vi "Host - 2954 - 6592R Tx Streaming.vi"() -> ()   [LabVIEW 2018, in "Stream-2954-6592R.lvlib"]
uses:
  Stream-2954-6592R.lvlib
  <vilib>/userDefined/Silver/nirio_resource_slv.ctl
  TypeDefs/USRP Configuration.ctl
  TypeDefs/Playback Options.ctl
  TypeDefs/TDMS read.ctl
  TDMS Raw to Channels/Previewed Channel - Enum.ctl
  TypeDefs/Tx Config.ctl
  2954/SubVIs/Start Trigger.ctl
  <instrlib>/niUsrpRio/Config/v1/Host/Public/niUsrpRio Session.ctl
  <instrlib>/_niInstr/Register Bus/v0/Host/Public/Register Bus Session.ctl
  <instrlib>/_niInstr/Register Bus/v0/Host/Private/Session Data.ctl
  <instrlib>/niUsrpRio/Config/v1/Host/Private/DB Queue Reference.ctl
  <instrlib>/niUsrpRio/Config/v1/Host/Private/Daughterboard Data.ctl
  <instrlib>/niUsrpRio/Config/v1/Host/Private/ATR state data.ctl
  <instrlib>/niUsrpRio/Config/v1/Host/Private/Antenna Configuration.ctl
  <instrlib>/niUsrpRio/Config/v1/Host/Private/CPLD Power Mode.ctl
  <instrlib>/niUsrpRio/Config/v1/Host/Public/EEPROM Header.ctl
  <instrlib>/niUsrpRio/Config/v1/Host/Public/EEPROM Device Data Header.ctl
  <instrlib>/niUsrpRio/Config/v1/Host/Public/EEPROM Characterization Header.ctl
  <instrlib>/niUsrpRio/Config/v1/Host/Public/Characterization Data.ctl
  <instrlib>/niUsrpRio/Config/v1/Host/Public/IQ Imbalance.ctl
  TypeDefs/Rx Config.ctl
  TypeDefs/States.ctl
  <vilib>/FPGAPlugInAG/Dynamic/niLvFpga_Close_Dynamic.vi
  <vilib>/rvi/interface/nirviCloseFPGA/nirviCloseFPGA.xnode
  <instrlib>/niUsrpRio/Config/v1/Host/niUsrpRio Config v1 Host.lvlib
  <instrlib>/_niInstr/Register Bus/v0/Host/niInstr Register Bus v0 Host.lvlib
panel:
  out "Generating":bool
  in  "Tab Control":enum32{"Settings", "Debug"}(tab)
  in  "Playback Options":T1={"Infinite Generation"=FALSE, "max asynch. reads"=8, "Samples per Write"=14000000, "chunks"=8, "disable buffering?"=TRUE} {"chunks" format="%.0p"; "Samples per Write" format="%.3p"}
  in  "TDMS file paths":path[](array[path])=[path "R:/USRP_recording_ch1.tdms", path "R:/USRP_recording_ch0.tdms"]
  out "Actual FIFO Depths":u32[][](array[numeric])=[[112000000, 112000000]] format="%.3p"
  out "Underflow":bool
  out "tx.number of fifo underflows":u32[](array[numeric])
  in  "tx config":T2={"rf enable 0"=TRUE, "rf config 0"={"antenna"="TX1", "frequency"=2000000000.0, "lo frequency"=-1.0, "level"=0.0}, "rf enable 1"=TRUE, "rf config 1"={"antenna"="TX1", "frequency"=2000000000.0, "lo frequency"=-1.0, "level"=0.0}, "transfer mode"=enum."Continuous", "sample rate"=200000000.0, "start trigger"=enum."Software"} {"sample rate" format="%#.3pS/s"; "rf config 0"."level" format="%#_gdBm"; "rf config 0"."lo frequency" format="%#.3pHz"; "rf config 0"."frequency" format="%#.3pHz"; "rf config 1"."level" format="%#_gdBm"; "rf config 1"."lo frequency" format="%#.3pHz"; "rf config 1"."frequency" format="%#.3pHz"}
  in  "USRP Configuration":T4={"USRP RIO Resources"=["USRP-2954_160MHz"], "reference frequency source"="Internal"}
  in  "6592R Resources":T5[](array[typedef])=["HSS"]
  in  "Previewed Channel":T6
  out "Channel progresses":dbl[](array[slide]) scale=0.0..100.0
  out "TDMS controls in":T7[][](array[typedef])=[[{"group name"="niRF", "channel name"="niRF_iq", "tdms file ref"=refnum, "file path"=path "R:/USRP record_ch1.tdms", "Channel Length"=914432000, "Number of reads"=65, "channel enabled"=TRUE}, {"group name"="niRF", "channel name"="niRF_iq", "tdms file ref"=refnum, "file path"=path "R:/USRP record_ch0.tdms", "Channel Length"=914432000, "Number of reads"=65, "channel enabled"=TRUE}]]
  in  "Exit":bool
  in  "Stop":bool
  in  "Run":bool
  out "Throughput (B/s)":dbl[](array[numeric])=[800000000.0, 800000000.0] format="%#.3p"
  out "Power Spectral Density (PSD)":cluster{"f0":dbl, "df":dbl, "magnitude":dbl[]}(graph)={"f0"=-100000000.0, "df"=100.0, "magnitude"=[]}
  # "Tx Aurora - 2 Channel Playback Demo"
  # "Throughput (B/s)"
  # "Recording Settings"
  # "Hardware Settings"
  # "Control Demo"
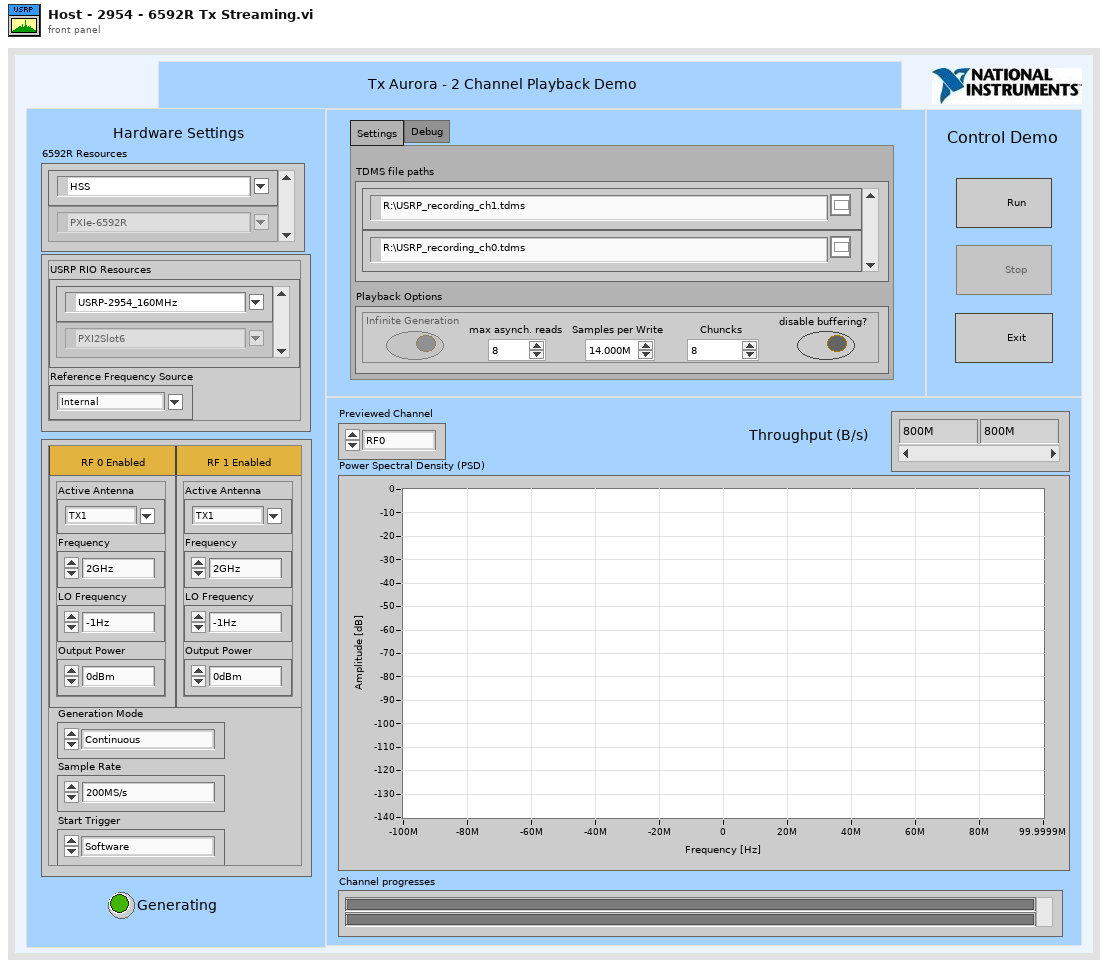
[diagram p1: front panel]
types:
  T1 = typedef "Playback Options.ctl" = cluster{"Infinite Generation":bool, "max asynch. reads":u32, "Samples per Write":u32, "chunks":u32, "disable buffering?":bool}
  T2 = typedef "Tx Config.ctl" = cluster{"rf enable 0":bool, "rf config 0":cluster{"antenna":string, "frequency":dbl, "lo frequency":dbl, "level":dbl}, "rf enable 1":bool, "rf config 1":cluster{"antenna":string, "frequency":dbl, "lo frequency":dbl, "level":dbl}, "transfer mode":enum16{"Finite", "Continuous"}, "sample rate":dbl, "start trigger":T3}
  T3 = typedef "Start Trigger.ctl" = enum8{"Software", "Digital Edge", "Rx Start Trigger", "Tx Start Trigger", "Immediate", "Future Time Event"}
  T4 = typedef "USRP Configuration.ctl" = cluster{"USRP RIO Resources":T5[], "reference frequency source":string}
  T5 = typedef "nirio_resource_slv.ctl" = tag
  T6 = typedef "Previewed Channel - Enum.ctl" = enum16{"RF0", "RF1"}
  T7 = typedef "TDMS read.ctl" = cluster{"group name":string, "channel name":string, "tdms file ref":refnum<k34>, "file path":path, "Channel Length":i64, "Number of reads":i64, "channel enabled":bool}
  T8 = typedef "niUsrpRio Config v1 Host.lvlib/niUsrpRio Session.ctl" = cluster{"FPGA Interface":refnum<k20>, "RIO Interface Number":u32, "Data Clock Rate":u32, "FPGA Data Clock Rate":u32, "Global Settings Register Bus":T9, "Radio 0 Settings Register Bus":T9, "Radio 1 Settings Register Bus":T9, "Radio Settings Bus Semaphore":T10, "DB Queues":T11[], "Characterization Data Valid?":bool, "EEPROM Header":T12, "Device Data Header":T13, "EEPROM Characterization Header":T14, "Characterization Data":T15[], "FPGA Current Version":u32, "FPGA Oldest Compatible Version":u32, "Fixed Logic Current Version":u32, "Fixed Logic Oldest Compatible Version":u32, "FPGA Radio Settings Bus Current Version":u32, "FPGA Radio Settings Bus Oldest Compatible Version":u32, "FPGA Board Config Current Version":u32, "FPGA Board Config Oldest Compatible Version":u32, "Daughterboard Clock Rate":u32, "daughterboard configuration session handles":u64[]}
  T9 = typedef "niInstr Register Bus v0 Host.lvlib/Register Bus Session.ctl" = refnum<queue>
  T10 = typedef "Semaphore RefNum" = refnum<k1>
  T11 = typedef "niUsrpRio Config v1 Host.lvlib/DB Queue Reference.ctl" = refnum<queue>
  T12 = typedef "niUsrpRio Config v1 Host.lvlib/EEPROM Header.ctl" = cluster{"Checksum":u32, "Product Code":u16, "Hardware Current Version":u16, "Hardware Oldest Compatible Version":u16, "EEPROM Map Current Version":u16, "EEPROM Map Oldest Compatible Version":u16, "User Password":string, "Pointer to Factory Header":u32, "Pointer to User Header":u32, "Recommended Interval":u16, "Number of Reserved Bytes":i32, "Number of Daughterboards":u8, "Daughterboard IDs":u16[], "Daughterboard Serial Numbers":string[]}
  T13 = typedef "niUsrpRio Config v1 Host.lvlib/EEPROM Device Data Header.ctl" = cluster{"Checksum":u32, "Number of Channels":u8, "Number of Gain Settings":u16[], "Pointer to Characterization Data":u32[], "Number of Reserved Bytes":i32, "Number of Frequencies":u16[]}
  T14 = typedef "niUsrpRio Config v1 Host.lvlib/EEPROM Characterization Header.ctl" = cluster{"Checksum":u32, "Date":timestamp, "Temperature":sgl, "Misc. Info":string, "Pointer to Device Data Header":u32, "Number of Reserved Bytes":i32}
  T15 = typedef "niUsrpRio Config v1 Host.lvlib/Characterization Data.ctl" = cluster{"Gains[dB]":dbl[], "Frequencies [Hz]":dbl[], "IQ Imbalance Table":T16[], "Measured Gains[dB]":dbl[][]}
  T16 = typedef "niUsrpRio Config v1 Host.lvlib/IQ Imbalance.ctl" = cluster{"Gain Imbalance [linear]":dbl, "Phase Imbalance [radians]":dbl, "Offset":cdb}
  T17 = typedef "Rx Config.ctl" = cluster{"rf enable 0":bool, "rf config 0":cluster{"antenna":string, "frequency":dbl, "lo frequency":dbl, "level":dbl}, "rf enable 1":bool, "rf config 1":cluster{"antenna":string, "frequency":dbl, "lo frequency":dbl, "level":dbl}, "transfer mode":enum16{"Finite", "Continuous"}, "sample rate":dbl, "start trigger":T3}
  T18 = cluster{"HS-Serial Resource":T5[], "USRP Configuration":T4, "File Path":path, "Refnum out":refnum<k20>[], "2 Ports?":bool[], "niUsrpRio Session":T8[], "Simulate Data?":bool, "TDMS Refnums out":refnum<k34>[], "rx config":T17, "TDMS controls in":T7[][], "Playback Options":T1, "tx config":T2}
  T19 = typedef "States.ctl" = enum16{"Choose Settings", "Exit", "Configure", "Run", "Close", "Shutdown", "transition to Run"}
  T20 = enum8{"Enabled", "Disabled", "Disabled and Grayed Out"}
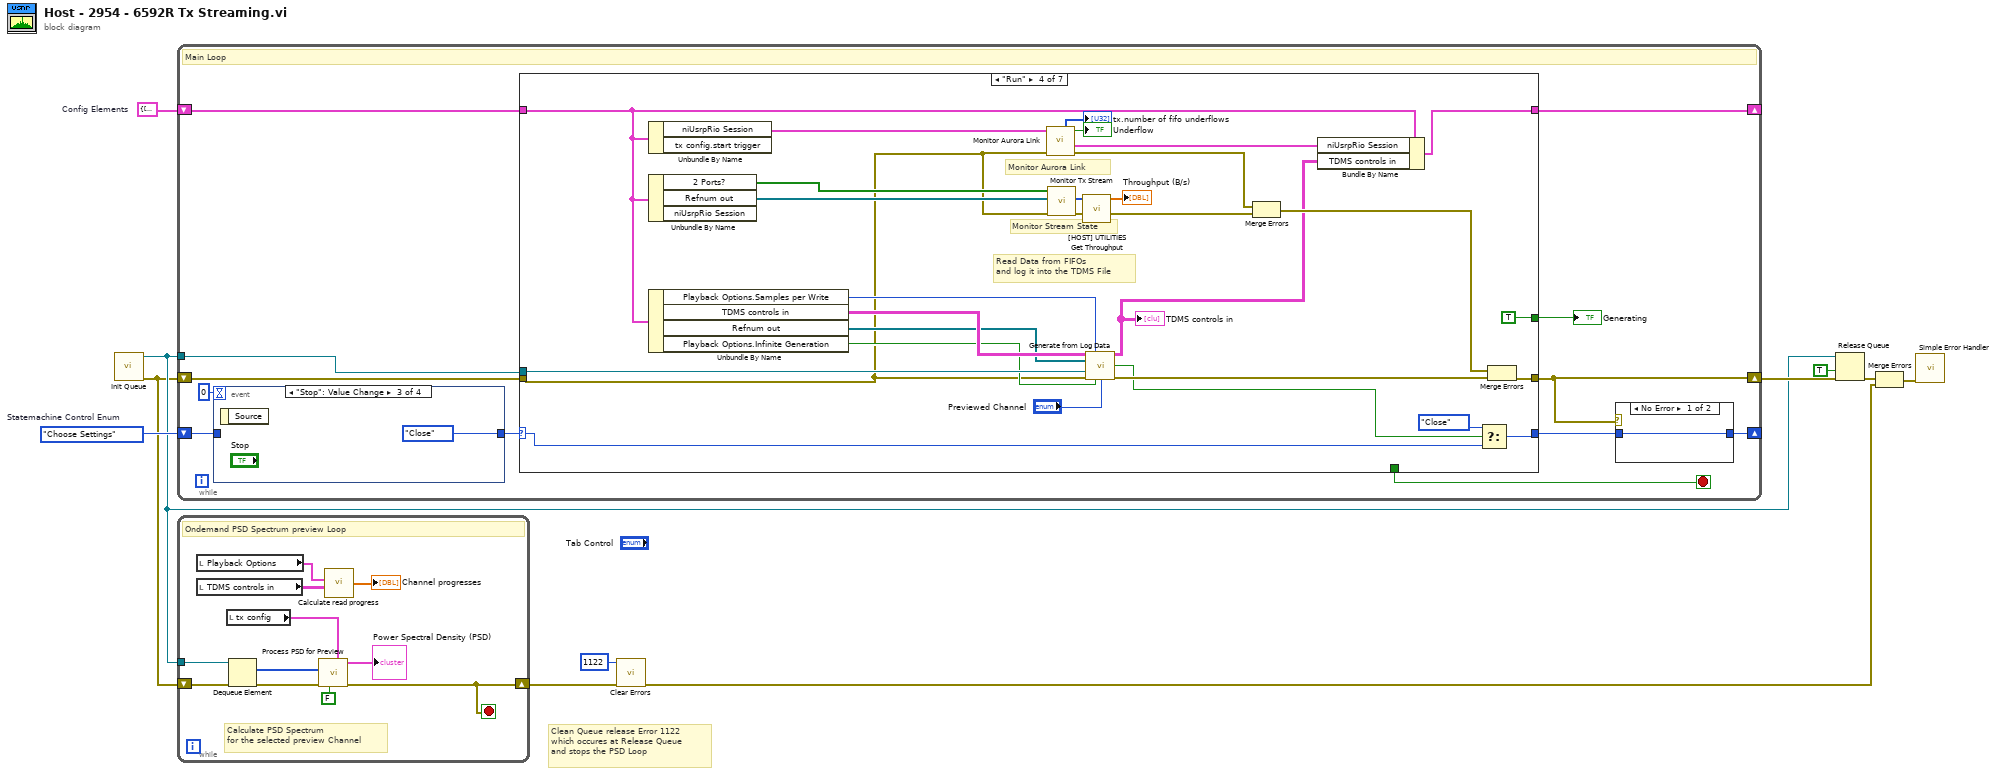
[diagram p0: block diagram]
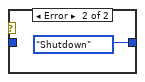
[diagram p2: hidden frame]
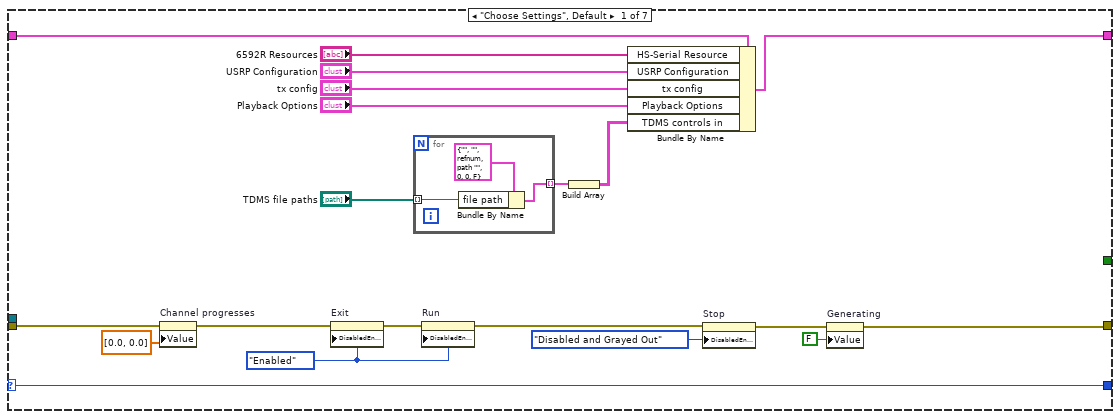
[diagram p3: hidden frame]
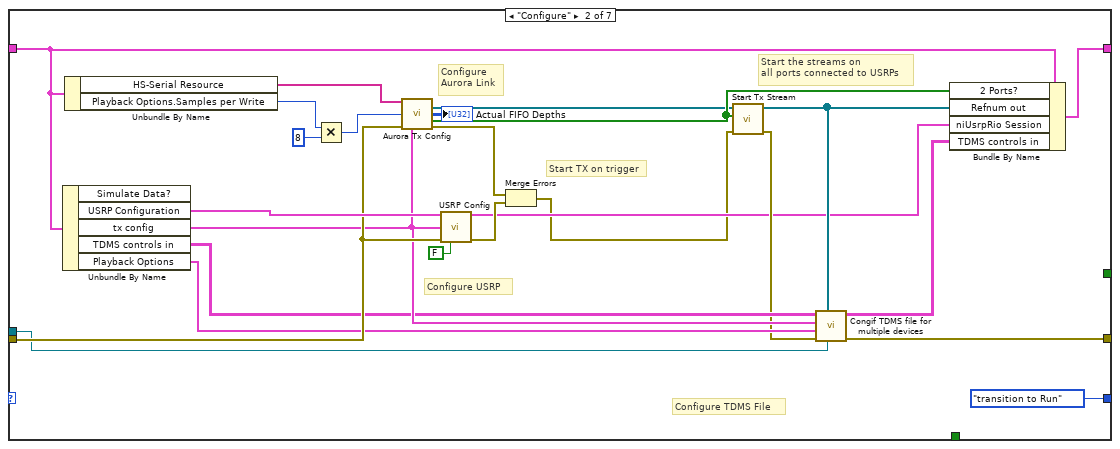
[diagram p4: hidden frame]
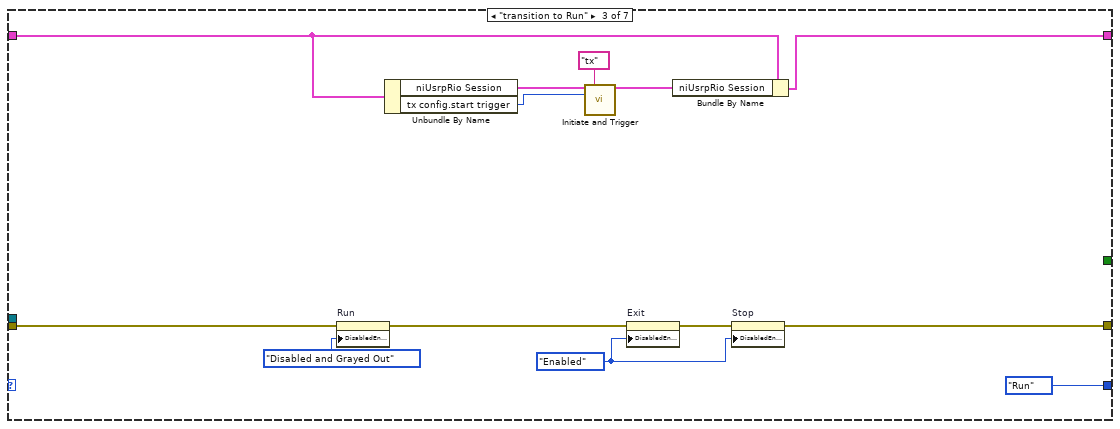
[diagram p5: hidden frame]
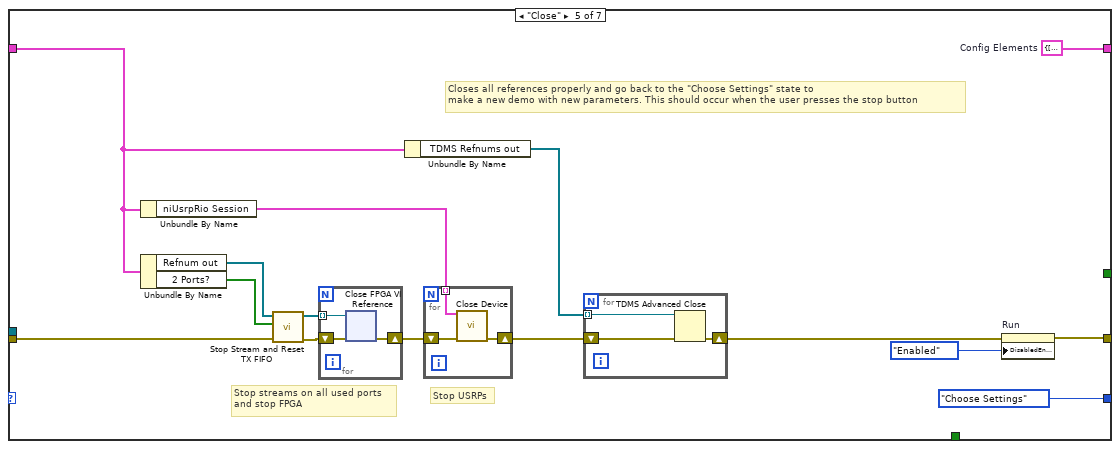
[diagram p6: hidden frame]
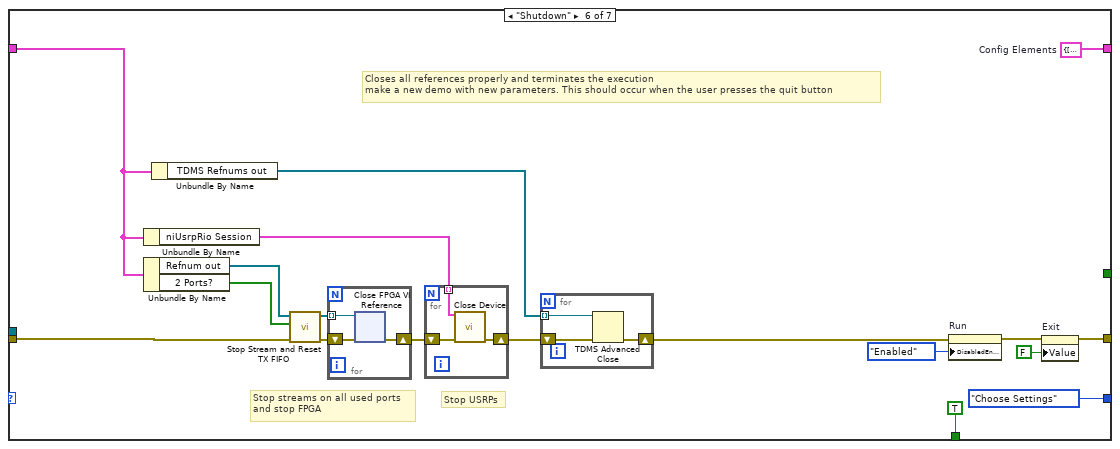
[diagram p7: hidden frame]
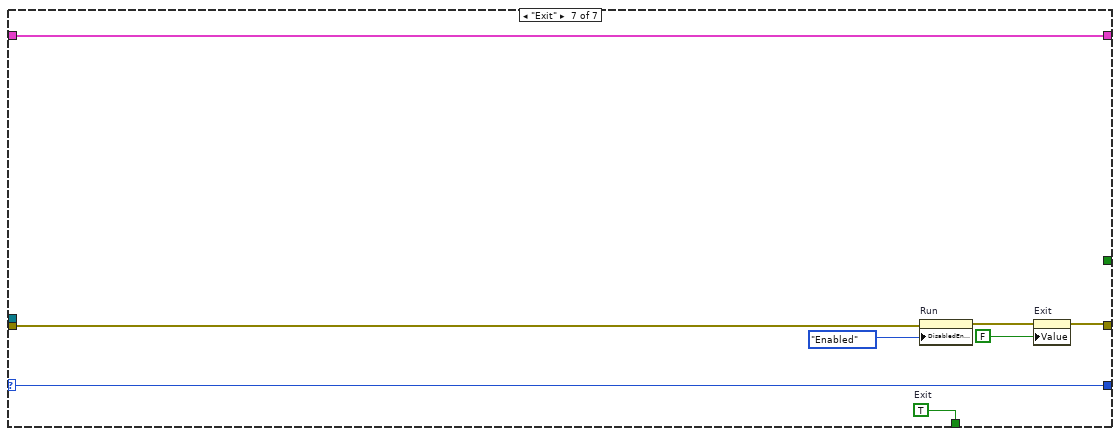
[diagram p8: hidden frame]
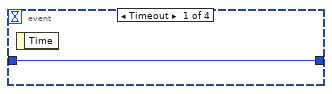
[diagram p9: hidden frame]
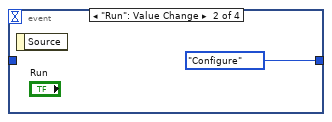
[diagram p10: hidden frame]
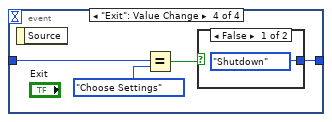
[diagram p11: hidden frame]
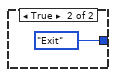
[diagram p12: hidden frame]
diagram:
  w1 = T18 {"HS-Serial Resource"=[], "USRP Configuration"={"USRP RIO Resources"=["USRP-2945"], "reference frequency source"="Internal"}, "File Path"=path "", "Refnum out"=[], "2 Ports?"=[], "niUsrpRio Session"=[], "Simulate Data?"=FALSE, "TDMS Refnums out"=[], "rx config"={"rf enable 0"=TRUE, "rf config 0"={"antenna"="RX2", "frequency"=2000000000.0, "lo frequency"=-1.0, "level"=0.0}, "rf enable 1"=TRUE, "rf config 1"={"antenna"="RX2", "frequency"=2000000000.0, "lo frequency"=-1.0, "level"=0.0}, "transfer mode"=enum."Finite", "sample rate"=10000000.0, "start trigger"=enum."Immediate"}, "TDMS controls in"=[], "Playback Options"={"Infinite Generation"=FALSE, "max asynch. reads"=8, "Samples per Write"=1024000, "chunks"=16, "disable buffering?"=FALSE}, "tx config"={"rf enable 0"=FALSE, "rf config 0"={"antenna"="TX1", "frequency"=2000000000.0, "lo frequency"=-1.0, "level"=0.0}, "rf enable 1"=FALSE, "rf config 1"={"antenna"="TX1", "frequency"=2000000000.0, "lo frequency"=-1.0, "level"=0.0}, "transfer mode"=enum."Finite", "sample rate"=10000000.0, "start trigger"=enum."Immediate"}}  # Config Elements
  w11 = States."Choose Settings"  # Statemachine Control Enum
  # "Clean Queue release Error 1122\nwhich occures at Release Queue \nand stops the PSD Loop"
  n1 = call "Init Queue.vi"() -> ("error out"=w4:errorcluster, "Queue out"=w5:refnum<queue>)  [unwired: 10 in]
  n2 = while {
    shift-right: [w17] -> _
    shift-left: w11 -> [w23]
    shift-right: [w16] -> w10
    shift-left: w4 -> [w20]
    shift-right: [w14] -> _
    shift-left: w1 -> [w15]
    tunnel: w5 -> [w13]
    stop <- w19 stop-if-true
    # "Main Loop"
    n3 = event shown="[2] \"Stop\": Value Change" {
      selector: _ -> [_ _ _ _]
      dyn-events: _ -> [_ _ _ _]
      timeout: 0 -> [_ _ _ _]
      tunnel: [w174 States."Configure" States."Close" w178] -> w22
      tunnel: w23 -> [w174 _ _ w179]
      event Timeout {
        n4 = event-data() -> ()  [unwired: 1 in, 1 out]
      }
      event "Run": Value Change {
        n5 = event-data() -> ()  [unwired: 1 in, 1 out]
      }
      event "Stop": Value Change {
        n6 = event-data() -> ()  [unwired: 1 in, 1 out]
      }
      event "Exit": Value Change {
        n7 = event-data() -> ()  [unwired: 1 in, 1 out]
        n8 = Equal?(x=w179, y=States."Choose Settings") -> (x = y?=w177:bool)
        n9 = case shown="False" w177 {
          tunnel: [States."Shutdown" States."Exit"] -> w178
          frame False {
          }
          frame True {
          }
        }
      }
    }
    n10 = case shown="\"Run\"" w22 {
      selector: w22 -> [w38 _ _ w98 _ _ w166]
      tunnel: [w26 w57 w85 w112 w125 w149 w170] -> w16
      tunnel: [w38 States."transition to Run" States."Run" w97 States."Choose Settings" States."Choose Settings" w166] -> w18
      tunnel: w20 -> [w32 w68 w83 w90 w117 w142 w167]
      tunnel: [_ _ _ _ _ TRUE w172] -> w19
      tunnel: w15 -> [w45 w70 w74 w113 w121 w153 w173]
      tunnel: [w43 w69 w75 w111 w115 w139 w173] -> w14
      tunnel: w13 -> [_ w55 _ w107 _ _ _]
      tunnel: [_ _ _ TRUE _ _ _] -> w12
      frame "Choose Settings", Default {
        w42 = T20."Enabled" ("Disabled")
        n11 = property on="Channel progresses" class="Arr (strict)"(error in=w32, "Value"=dbl[] [0.0, 0.0] ("Read percentages")) -> (error out=w31:errorcluster)  [unwired: 1 in, 1 out]
        n12 = property on="Exit" class="Bool (strict)"(error in=w31, "DisabledEnum"=w42) -> (error out=w41:errorcluster)  [unwired: 1 in, 1 out]
        n13 = for {
          tunnel: "TDMS file paths" -> [w47] mode=indexing
          tunnel: [w48] -> w34 mode=indexing
          n14 = Bundle By Name(cluster=T7 {"group name"="", "channel name"="", "tdms file ref"=refnum, "file path"=path "", "Channel Length"=0, "Number of reads"=0, "channel enabled"=FALSE} ("TDMS read controls in"), "file path"=w47) -> (w48:T7)
        }
        n15 = property on="Run" class="Bool"(error in=w41, "DisabledEnum"=w42) -> (error out=w40:errorcluster)  [unwired: 1 in, 1 out]
        n16 = Build Array(w34) -> (w35:T7[][])
        n17 = Bundle By Name(cluster=w45, "HS-Serial Resource"="6592R Resources", "USRP Configuration"="USRP Configuration", "tx config"="tx config", "Playback Options"="Playback Options", "TDMS controls in"=w35) -> (w43:T18)
        n18 = property on="Stop" class="Bool"(error in=w40, "DisabledEnum"=T20."Disabled and Grayed Out" ("Disabled")) -> (error out=w28:errorcluster)  [unwired: 1 in, 1 out]
        n19 = property on="Generating" class="Bool (strict)"(error in=w28, "Value"=FALSE ("Generating")) -> (error out=w26:errorcluster)  [unwired: 1 in, 1 out]
      }
      frame "Configure" {
        # "Start TX on trigger"
        # "Configure USRP"
        # "Configure TDMS File"
        # "Start the streams on \nall ports connected to USRPs"
        # "Configure \nAurora Link"
        n20 = Unbundle By Name(w70) -> ("USRP Configuration"=w72:T4, "tx config"=w65:T2, "TDMS controls in"=w64:T7[][], "Playback Options"=w60:T1)  [unwired: 1 out]
        n21 = Unbundle By Name(w70) -> ("HS-Serial Resource"=w71:T5[], "Playback Options.Samples per Write"=w52:u32)
        n22 = Multiply(x=w52, y=u32 8) -> (x*y=w50:u32)
        n23 = call "Aurora Tx Config.vi"("6592R Resources"=w71, "FIFO Depth"=w50, "error in (no error)"=w68, "tx config"=w65) -> ("Refnum out"=w61:refnum<k20>[], "Actual FIFO Depths"=→"Actual FIFO Depths":u32[][], "2 Ports?"=w62:bool[], "error out"=w67:errorcluster)  [unwired: 7 in, 1 out]
        n24 = call "USRP Config.vi"("USRP Configuration"=w72, "tx config"=w65, "error in (no error)"=w68, "Rx?"=FALSE) -> ("niUsrpRio Session"=w54:T8[], "error out"=w63:errorcluster)  [unwired: 3 in, 7 out]
        n25 = Merge Errors(w67, w63) -> (w53:errorcluster)
        n26 = call "Start Tx Stream.vi"("error in (no error)"=w53, "2 Ports?"=w62, "Refnum in"=w61) -> ("error out"=w58:errorcluster, "Refnum out"=w56:refnum<k20>[])  [unwired: 7 in]
        n27 = call "Congif TDMS file for multiple devices.vi"("Queue in"=w55, "HSS Resource references"=w56, "error in (no error)"=w58, "Playback Options"=w60, "tx config"=w65, "TDMS controls in"=w64) -> ("error out"=w57:errorcluster, "TDMS read controls out"=w66:T7[][])  [unwired: 4 in]
        n28 = Bundle By Name(cluster=w70, "2 Ports?"=w62, "Refnum out"=w56, "niUsrpRio Session"=w54, "TDMS controls in"=w66) -> (w69:T18)
      }
      frame "transition to Run" {
        w84 = T20."Enabled" ("Disabled")
        n29 = property on="Run" class="Bool"(error in=w83, "DisabledEnum"=T20."Disabled and Grayed Out" ("Disabled")) -> (error out=w82:errorcluster)  [unwired: 1 in, 1 out]
        n30 = Unbundle By Name(w74) -> ("niUsrpRio Session"=w79:T8[], "tx config.start trigger"=w78:T3)
        n31 = call "Initiate and Trigger.vi"("niUsrpRio Sessions"=w79, "scope"="tx", "start trigger"=w78) -> ("niUsrpRio Sessions (out)"=w76:T8[])  [unwired: 11 in, 1 out]
        n32 = property on="Exit" class="Bool (strict)"(error in=w82, "DisabledEnum"=w84) -> (error out=w86:errorcluster)  [unwired: 1 in, 1 out]
        n33 = Bundle By Name(cluster=w74, "niUsrpRio Session"=w76) -> (w75:T18)
        n34 = property on="Stop" class="Bool"(error in=w86, "DisabledEnum"=w84) -> (error out=w85:errorcluster)  [unwired: 1 in, 1 out]
      }
      frame "Run" {
        # "Monitor Aurora Link"
        # "Read Data from FIFOs \nand log it into the TDMS File"
        # "Monitor Stream State"
        n35 = Unbundle By Name(w113) -> ("niUsrpRio Session"=w89:T8[])  [unwired: 1 out]
        n36 = Unbundle By Name(w113) -> ("2 Ports?"=w101:bool[], "Refnum out"=w93:refnum<k20>[])  [unwired: 1 out]
        n37 = Unbundle By Name(w113) -> ("Playback Options.Samples per Write"=w102:u32, "TDMS controls in"=w106:T7[][], "Refnum out"=w105:refnum<k20>[], "Playback Options.Infinite Generation"=w104:bool)
        n38 = call "Monitor Aurora Link.vi"("error in (no error)"=w90, "niUsrpRio Sessions (In)"=w89) -> ("error out"=w110:errorcluster, "niUsrpRio Sessions (Out)"=w108:T8[], "underflow"=→"Underflow":bool, "tx.number of fifo underflows"=→"tx.number of fifo underflows":u32[])  [unwired: 5 in, 1 out]
        n39 = call "Monitor Tx Stream.vi"("error in (no error)"=w90, "Refnum in"=w93, "2 USRPs?"=w101) -> ("error out"=w99:errorcluster, "Samples Transferred"=w100:u64[])  [unwired: 6 in, 1 out]
        n40 = call "[HOST] UTILITIES Get Throughput.vi"("Samples"=w100) -> ("Throughput"=→"Throughput (B/s)":dbl[])  [unwired: 10 in]
        n41 = call "Generate from Log Data.vi"("TDMS controls in"=w106, "Samples per Write"=w102, "HSS Resource references"=w105, "Queue in"=w107, "error in"=w90, "Infinite Gene"=w104, "Previewed Channel"="Previewed Channel") -> ("TDMS controls out"=w95:T7[][], "Asynchronous \nRead Finished?"=w87:bool, "error out"=w103:errorcluster)  [unwired: 3 in, 3 out]
        "TDMS controls in" <- w95
        n42 = Merge Errors(w110, w99) -> (w109:errorcluster)
        n43 = Bundle By Name(cluster=w113, "niUsrpRio Session"=w108, "TDMS controls in"=w95) -> (w111:T18)
        n44 = Select(t=States."Close", s=w87, f=w98) -> (s? t:f=w97:T19)
        n45 = Merge Errors(w109, w103) -> (w112:errorcluster)
      }
      frame "Close" {
        w115 = T18 {"HS-Serial Resource"=[], "USRP Configuration"={"USRP RIO Resources"=["USRP-2945"], "reference frequency source"="Internal"}, "File Path"=path "", "Refnum out"=[], "2 Ports?"=[], "niUsrpRio Session"=[], "Simulate Data?"=FALSE, "TDMS Refnums out"=[], "rx config"={"rf enable 0"=TRUE, "rf config 0"={"antenna"="RX2", "frequency"=2000000000.0, "lo frequency"=-1.0, "level"=0.0}, "rf enable 1"=TRUE, "rf config 1"={"antenna"="RX2", "frequency"=2000000000.0, "lo frequency"=-1.0, "level"=0.0}, "transfer mode"=enum."Finite", "sample rate"=10000000.0, "start trigger"=enum."Immediate"}, "TDMS controls in"=[], "Playback Options"={"Infinite Generation"=FALSE, "max asynch. reads"=8, "Samples per Write"=1024000, "chunks"=16, "disable buffering?"=FALSE}, "tx config"={"rf enable 0"=FALSE, "rf config 0"={"antenna"="TX1", "frequency"=2000000000.0, "lo frequency"=-1.0, "level"=0.0}, "rf enable 1"=FALSE, "rf config 1"={"antenna"="TX1", "frequency"=2000000000.0, "lo frequency"=-1.0, "level"=0.0}, "transfer mode"=enum."Finite", "sample rate"=10000000.0, "start trigger"=enum."Immediate"}}  # Config Elements
        # "Closes all references properly and go back to the \"Choose Settings\" state to \nmake a new demo with new parameters. This should occur when the user presses the stop button"
        # "Stop streams on all used ports \nand stop FPGA"
        # "Stop USRPs"
        n46 = Unbundle By Name(w121) -> ("niUsrpRio Session"=w127:T8[])
        n47 = Unbundle By Name(w121) -> ("Refnum out"=w119:refnum<k20>[], "2 Ports?"=w118:bool[])
        n48 = call "Stop Stream and Reset TX FIFO.vi"("error in (no error)"=w117, "2 USRPs?"=w118, "Refnum in"=w119) -> ("error out"=w116:errorcluster, "Refnum out"=w120:refnum<k20>[])  [unwired: 7 in]
        n49 = for {
          tunnel: w120 -> [w137] mode=indexing
          shift-right: [w138] -> w129
          shift-left: w116 -> [w136]
          n50 = xnode "Close FPGA VI Reference"("FPGA VI Reference In"=w137, "error in"=w136) -> ("error out"=w138:errorcluster)
        }
        n51 = Unbundle By Name(w121) -> ("TDMS Refnums out"=w124:refnum<k34>[])
        n52 = for {
          shift-right: [w134] -> w123
          shift-left: w129 -> [w135]
          tunnel: w127 -> [w133] mode=indexing
          n53 = call "Close Device.vi"("niUsrpRio Session"=w133, "error in"=w135) -> ("error out"=w134:errorcluster)  [unwired: 13 in]
        }
        n54 = for {
          shift-right: [w131] -> w122
          shift-left: w123 -> [w132]
          tunnel: w124 -> [w130] mode=indexing
          n55 = TDMS Advanced Close(8:w132, 11:w130) -> (0:w131:errorcluster)  [unwired: 2 in, 1 out]
        }
        n56 = property on="Run" class="Bool"(error in=w122, "DisabledEnum"=T20."Enabled" ("Disabled")) -> (error out=w125:errorcluster)  [unwired: 1 in, 1 out]
      }
      frame "Shutdown" {
        w139 = T18 {"HS-Serial Resource"=[], "USRP Configuration"={"USRP RIO Resources"=["USRP-2945"], "reference frequency source"="Internal"}, "File Path"=path "", "Refnum out"=[], "2 Ports?"=[], "niUsrpRio Session"=[], "Simulate Data?"=FALSE, "TDMS Refnums out"=[], "rx config"={"rf enable 0"=TRUE, "rf config 0"={"antenna"="RX2", "frequency"=2000000000.0, "lo frequency"=-1.0, "level"=0.0}, "rf enable 1"=TRUE, "rf config 1"={"antenna"="RX2", "frequency"=2000000000.0, "lo frequency"=-1.0, "level"=0.0}, "transfer mode"=enum."Finite", "sample rate"=10000000.0, "start trigger"=enum."Immediate"}, "TDMS controls in"=[], "Playback Options"={"Infinite Generation"=FALSE, "max asynch. reads"=8, "Samples per Write"=1024000, "chunks"=16, "disable buffering?"=FALSE}, "tx config"={"rf enable 0"=FALSE, "rf config 0"={"antenna"="TX1", "frequency"=2000000000.0, "lo frequency"=-1.0, "level"=0.0}, "rf enable 1"=FALSE, "rf config 1"={"antenna"="TX1", "frequency"=2000000000.0, "lo frequency"=-1.0, "level"=0.0}, "transfer mode"=enum."Finite", "sample rate"=10000000.0, "start trigger"=enum."Immediate"}}  # Config Elements
        # "Stop streams on all used ports \nand stop FPGA"
        # "Closes all references properly and terminates the execution\nmake a new demo with new parameters. This should occur when the user presses the quit button"
        # "Stop USRPs"
        n57 = Unbundle By Name(w153) -> ("niUsrpRio Session"=w154:T8[])
        n58 = Unbundle By Name(w153) -> ("Refnum out"=w144:refnum<k20>[], "2 Ports?"=w143:bool[])
        n59 = Unbundle By Name(w153) -> ("TDMS Refnums out"=w147:refnum<k34>[])
        n60 = call "Stop Stream and Reset TX FIFO.vi"("error in (no error)"=w142, "2 USRPs?"=w143, "Refnum in"=w144) -> ("error out"=w141:errorcluster, "Refnum out"=w140:refnum<k20>[])  [unwired: 7 in]
        n61 = for {
          tunnel: w140 -> [w164] mode=indexing
          shift-right: [w165] -> w156
          shift-left: w141 -> [w163]
          n62 = xnode "Close FPGA VI Reference"("FPGA VI Reference In"=w164, "error in"=w163) -> ("error out"=w165:errorcluster)
        }
        n63 = for {
          shift-right: [w161] -> w146
          shift-left: w156 -> [w162]
          tunnel: w154 -> [w160] mode=indexing
          n64 = call "Close Device.vi"("niUsrpRio Session"=w160, "error in"=w162) -> ("error out"=w161:errorcluster)  [unwired: 13 in]
        }
        n65 = for {
          shift-right: [w158] -> w145
          shift-left: w146 -> [w159]
          tunnel: w147 -> [w157] mode=indexing
          n66 = TDMS Advanced Close(8:w159, 11:w157) -> (0:w158:errorcluster)  [unwired: 2 in, 1 out]
        }
        n67 = property on="Run" class="Bool"(error in=w145, "DisabledEnum"=T20."Enabled" ("Disabled")) -> (error out=w148:errorcluster)  [unwired: 1 in, 1 out]
        n68 = property on="Exit" class="Bool (strict)"(error in=w148, "Value"=FALSE ("Exit")) -> (error out=w149:errorcluster)  [unwired: 1 in, 1 out]
      }
      frame "Exit" {
        w172 = TRUE  # Exit
        n69 = property on="Run" class="Bool"(error in=w167, "DisabledEnum"=T20."Enabled" ("Disabled")) -> (error out=w168:errorcluster)  [unwired: 1 in, 1 out]
        n70 = property on="Exit" class="Bool (strict)"(error in=w168, "Value"=FALSE ("Exit")) -> (error out=w170:errorcluster)  [unwired: 1 in, 1 out]
      }
    }
    "Generating" <- w12
    n71 = case shown="No Error" w16 {
      tunnel: [w24 States."Shutdown"] -> w17
      tunnel: w18 -> [w24 _]
      frame No Error {
      }
      frame Error {
      }
    }
  }
  n72 = while {
    shift-right: [w188] -> w6
    shift-left: w4 -> [w193]
    tunnel: w5 -> [w191]
    stop <- w188 stop-if-true
    # "Calculate PSD Spectrum\nfor the selected preview Channel"
    # "Ondemand PSD Spectrum preview Loop"
    n73 = local read "Playback Options"() -> (w184:T1)
    n74 = local read "TDMS controls in"() -> (w185:T7[][])
    n75 = local read "tx config"() -> (w187:T2)
    n76 = Dequeue Element(queue=w191, error in (no error)=w193) -> (element=w189:u64[], error out=w192:errorcluster)  [unwired: 1 in, 2 out]
    n77 = call "Process PSD for Preview.vi"("tx config"=w187, "Rx?"=FALSE, "error in (no error)"=w192, "Data Array"=w189) -> ("error out"=w188:errorcluster, "Power Spectrum / PSD"=→"Power Spectral Density (PSD)":cluster{"f0":dbl, "df":dbl, "magnitude":dbl[]})  [unwired: 6 in]
    n78 = call "Calculate read progress.vi"("TDMS controls in"=w185, "Playback Options"=w184) -> ("Read progress [%]"=→"Channel progresses":dbl[])  [unwired: 4 in]
  }
  n79 = call <vilib>:"Clear Errors.vi"("error in (no error)"=w6, "specific error code to clear (0: all)"=1122) -> ("error out"=w3:errorcluster)  [unwired: 4 in, 1 out]
  n80 = Release Queue(queue=w5, force destroy? (F)=TRUE, error in (no error)=w10) -> (error out=w8:errorcluster)  [unwired: 2 out]
  n81 = Merge Errors(w8, w3) -> (w7:errorcluster)
  n82 = call <vilib>:"Simple Error Handler.vi"("error in (no error)"=w7) -> ()  [unwired: 4 in, 5 out]
